vi "Get VI Infomation.vi"(8 "error in (no error)":errorcluster, 11 "Model in":refnum<class "Model.lvclass">) -> (0 "error out":errorcluster, 3 "Model out":refnum<class "Model.lvclass">)   [LabVIEW 2015, in "Model.lvlib" / "Model.lvclass"]
uses:
  Model.lvclass
  Controls/VI Infomation.ctl
  Model.lvlib
  Interface Messages/Update VI List Msg/Update VI List Msg.lvclass
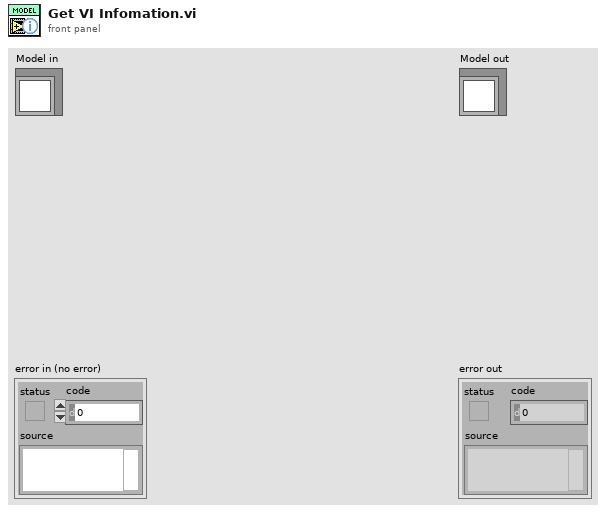
[diagram p1: front panel]
types:
  T1 = typedef "Model.lvlib/VI Infomation.ctl" = cluster{"Name":string, "Description":string, "Icon":picture}
  T2 = typedef "imagedata.ctl" = cluster{"image type":i32, "image depth":i32, "image":u8[], "mask":u8[], "colors":u32[], "Rectangle":cluster{"left":i16, "top":i16, "right":i16, "bottom":i16}}
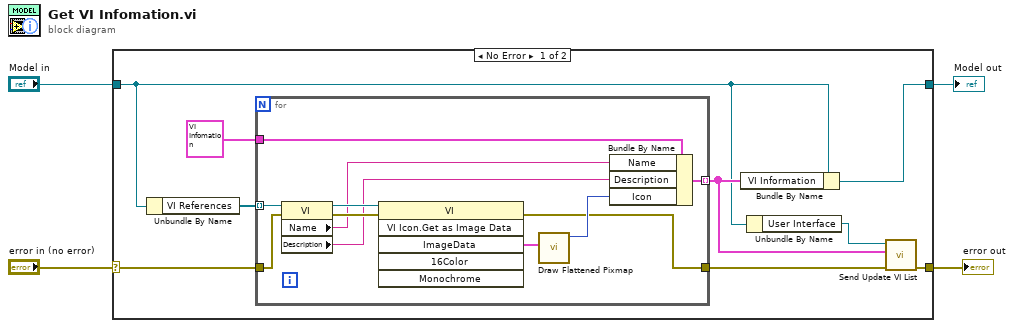
[diagram p0: block diagram]
diagram:
  n1 = case shown="No Error" "error in (no error)" {
    selector: "error in (no error)" -> [w12 w26]
    tunnel: [w7 w26] -> w3
    tunnel: [w11 w25] -> w1
    tunnel: "Model in" -> [w6 w25]
    frame No Error {
      n2 = Unbundle By Name(w6) -> ("VI References"=w13:refnum<vi>[])
      n3 = for {
        tunnel: w13 -> [w23] mode=indexing
        tunnel: w12 -> [w20]
        tunnel: T1 {"Name"="", "Description"="", "Icon"=bytes[0]} ("VI Infomation") -> [w19]
        tunnel: [w15] -> w9 mode=indexing
        tunnel: [w14] -> w8
        n4 = property class="VI"(reference=w23, error in=w20) -> (reference out=w22:refnum<vi>, error out=w21:errorcluster, "Name"=w18:string, "Description"=w17:string)
        n5 = invoke class="VI" method="VI Icon.Get as Image Data"(reference=w22, error in=w21) -> (error out=w14:errorcluster, "ImageData"=w24:T2)  [unwired: 4 in, 4 out]
        n6 = call <vilib>:"Draw Flattened Pixmap.vi"("image data"=w24) -> ("new picture"=w16:picture)  [unwired: 8 in]
        n7 = Bundle By Name(cluster=w19, "Name"=w18, "Description"=w17, "Icon"=w16) -> (w15:T1)
      }
      n8 = Bundle By Name(cluster=w6, "VI Information"=w9) -> (w11:refnum<class "Model.lvclass">)
      n9 = Unbundle By Name(w6) -> ("User Interface"=w5:refnum<class "Message Enqueuer.lvclass">)
      n10 = call "Send Update VI List.vi"("error in (no error)"=w8, "VI Infomation"=w9, "Message Enqueuer"=w5) -> ("error out"=w7:errorcluster)  [unwired: 7 in, 1 out]
    }
    frame Error {
    }
  }
  "error out" <- w3
  "Model out" <- w1
